vi "Speak text ASYNC.vi"(2 "Text to speak":string="Warning, Allan Wells will give you a thick ear. Please proceed with caution.") -> (0 "error out":errorcluster)   [LabVIEW 2013]
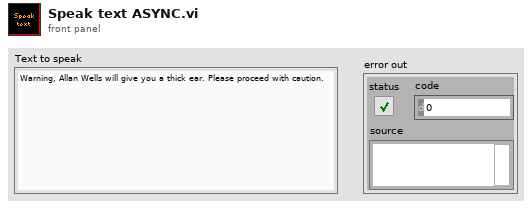
[diagram p1: front panel]
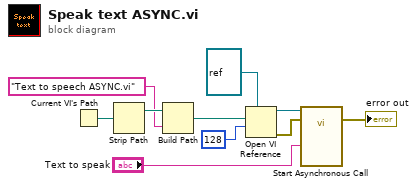
[diagram p0: block diagram]
diagram:
  n1 = Current VI's Path() -> (path=w4:path)
  n2 = Strip Path(path=w4) -> (stripped path=w3:path)  [unwired: 1 out]
  n3 = Build Path(base path=w3, name or relative path="Text to speech ASYNC.vi") -> (appended path=w2:path)
  n4 = Open VI Reference(type specifier VI Refnum (for type only)=refnum<vi> refnum, vi path=w2, options=128) -> (vi reference=w9:refnum<vi>, error out=w8:errorcluster)  [unwired: 3 in]
  n5 = call-by-ref "Start Asynchronous Call"(reference=w9, error in=w8, "Text to speak"="Text to speak") -> (error out=→"error out":errorcluster)  [unwired: 1 out]
